vi "zlgcan_demo_I.vi"() -> ()   [LabVIEW 2013]
doc: "适用的设备：USBCAN-I、USBCAN-II、PCI9810、\nPCI9820、PCI5110、PCIe-9110I、PCI9820I、PCIE-9221、\nPCIe-9120I、PCI5121。"
uses:
  data_type/ZCAN_Transmit_Data.ctl
  data_type/ZCAN_InitCAN_setting_I.ctl
panel:
  in  "开启CAN":bool
  in  "I系列初始化参数":T1
  in  "stop":bool
  in  "?":T2(tab)
  in  "CAN 通道":u32(ring) items=["0", "1"]
  in  "CAN卡型号":u32(ring)=4 items=["PCI5121"=1, "PCI9810"=2, "USBCAN-I"=3, "USBCAN-II"=4, "PCI9820"=5, "PCI5110"=7, "CANET-UDP"=12, "PCI9840B"=14, "PCI9820I"=16, "CANET-TCP"=17, "PCIE9221"=24, "PCI-5010-U"=19, "PCI-5020-U"=22, "USBCAN_E_U"=20, "USBCAN_2E_U"=21, "USBCAN-4E-U"=31, "USBCAN-8E-U"=34, "PCIE-CANFD-400U"=40, "PCIE-CANFD-200U"=39, "PCIE-CANFD-100U"=38, "USBCANFD-200U"=41, "USBCANFD-100U"=42, "USBCANFD-MINI"=43, "PCIE-9120I"=27, "PCIE-9110I"=28, "PCIE-9140I"=29, "CANDTU-MINI"=33, "CANDTU-200 XX"=32]
  in  "索引":u32(ring) items=["0", "1", "2", "3", "4", "5", "6", "7", "8"]
  in  "波特率":u32(ring)=500000 items=["1Mbps"=1000000, "800kbps"=800000, "500kbps"=500000, "250kbps"=250000, "125kbps"=125000, "100kbps"=100000, "50kbps"=50000]
  in  "自定义波特率？":bool
  in  "自定义波特率字符输入":string
  in  "屏蔽码":u32=4294967295 format="%x"
  in  "工作模式":u8(ring) items=["正常", "只听"]
  in  "滤波模式":u8(ring) items=["双滤波", "单滤波"]
  in  "验收码":u32
  out "设备句柄":u32
  out "通道句柄":u32
  out "error out":errorcluster caption="状态"
  in  "帧类型":u32(ring) items=["标准帧", "扩展帧"]
  in  "发送方式":u32(ring) items=["正常发送", "单次发送", "自发自收", "单次自发自收"]
  in  "帧格式":u32(ring) items=["数据帧", "远程帧"]
  out "数据长度":u8=8 max=8
  in  "ID":u32=18 format="0x%08x"
  in  "协议":u32(ring) items=["CAN"]
  in  "数据输入":string="11 22 33 44 55 66 77 88"
  in  "发送":bool
  in  "CAN数据帧数组":T3(array[cluster])
  out "CAN报文显示":string[][](table)
  in  "ZCAN_Transmit_Data":T4
  out "已接收帧数":u32
  # "适用的设备：USBCAN-I、USBCAN-II、PCI9810、\nPCI9820、PCI5110、PCIe-9110I、PCI9820I、PCIE-9221、\nPCIe-9120I、PCI5121。"
  # "停止程序前，\n请先关闭CAN卡"
  # "1. 调试运行DEMO前，将bin文件夹下面的kerneldlls文件夹先拷贝至LabView安装目录，\n如 D:\\Program Files (x86)\\National Instruments\\LabVIEW 2018。"
  # "2. 确保电脑有VC++ 2005/2008/2010/2013运行库（对应32，64位），可到微软官网下载。"
  # "3，如果打开设备失败，可能原因：\n（1）没有进行第二步操作；\n（2）已经打开过一次，没有正常关闭的情况下，继续点击“打开设备”，是无法打开的。\n     需要USB重新拔插，LABVIEW重启（全部关闭），然后再“打开设备”。\n (3) 项目路径不能有中文繁体。"
  # "（默认可以不设置）"
  # "使用ZCANPro软件波特率计算工具计算"
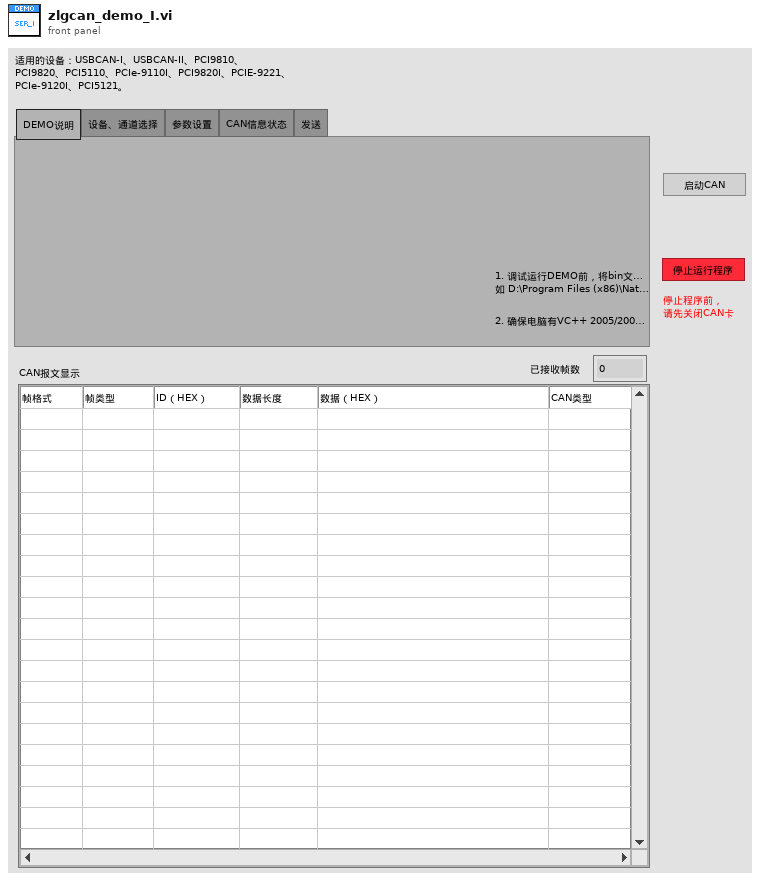
[diagram p1: front panel]
types:
  T1 = typedef "ZCAN_InitCAN_setting_I.ctl" = cluster{"baudrate":u32, "baud_rate_custom？":bool, "RateCustom":string, "filter":u8, "acc_code":u32, "acc_mask":u32, "mode":u8}
  T2 = enum32{"DEMO说明", "设备、通道选择", "参数设置", "CAN信息状态", "发送"}
  T3 = cluster{u32, u8, u8, u8, u8, cluster{"[0]":u8, "[1]":u8, "[2]":u8, "[3]":u8, "[4]":u8, "[5]":u8, "[6]":u8, "[7]":u8}, u64}[]
  T4 = typedef "ZCAN_Transmit_Data.ctl" = cluster{"帧类型":u32, "帧格式":u32, "ID":u32, "数据长度":u8, "DATA":cluster{"CAN数据[0]":u8, "CAN数据[1]":u8, "CAN数据[2]":u8, "CAN数据[3]":u8, "CAN数据[4]":u8, "CAN数据[5]":u8, "CAN数据[6]":u8, "CAN数据[7]":u8}, "发送方式":u32}
  T5 = cluster{"[0]":u32, "[1]":u32, "[2]":u32, "[3]":u32, "[4]":u32, "[5]":u32, "[6]":u32, "[7]":u32}
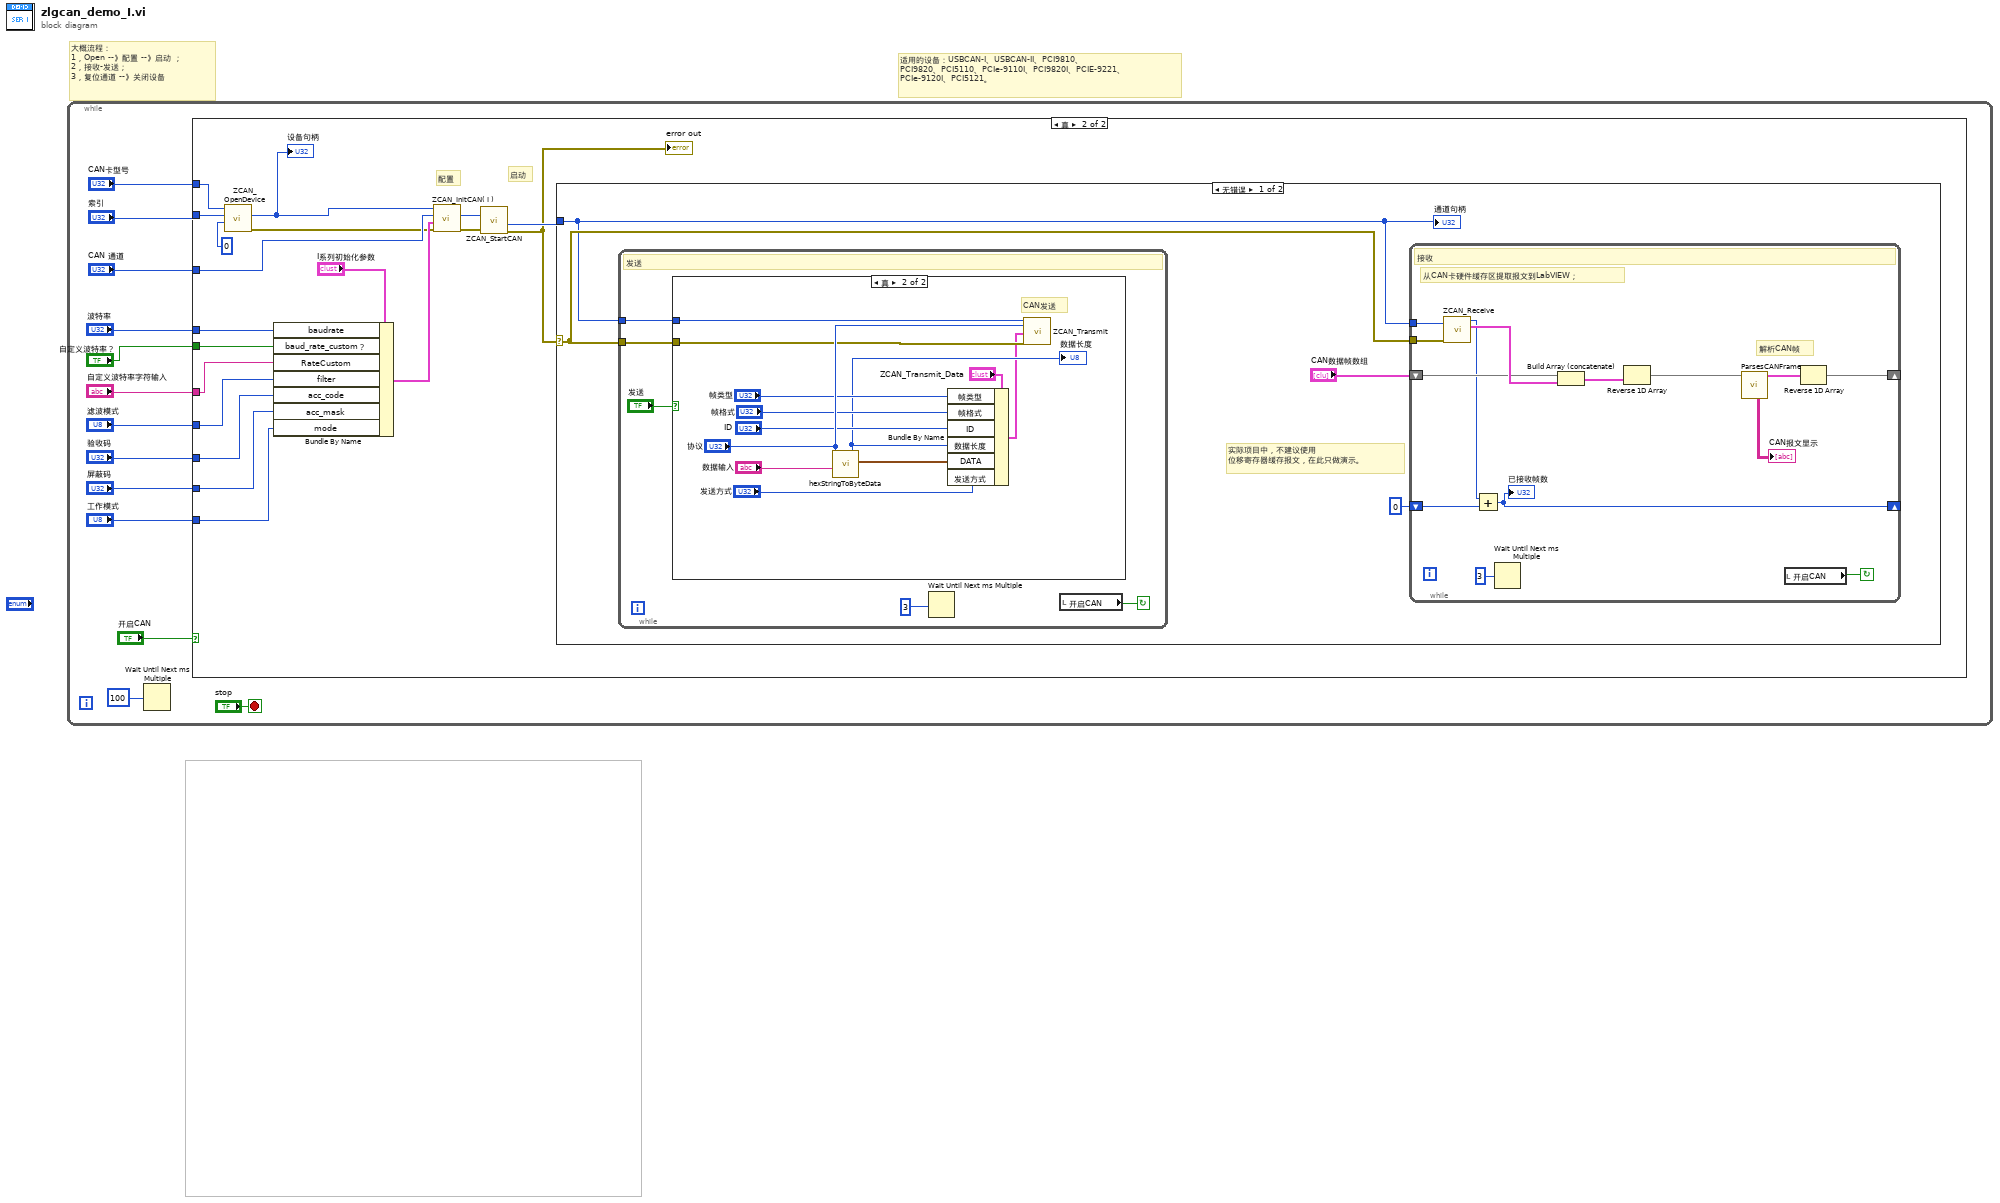
[diagram p0: block diagram]
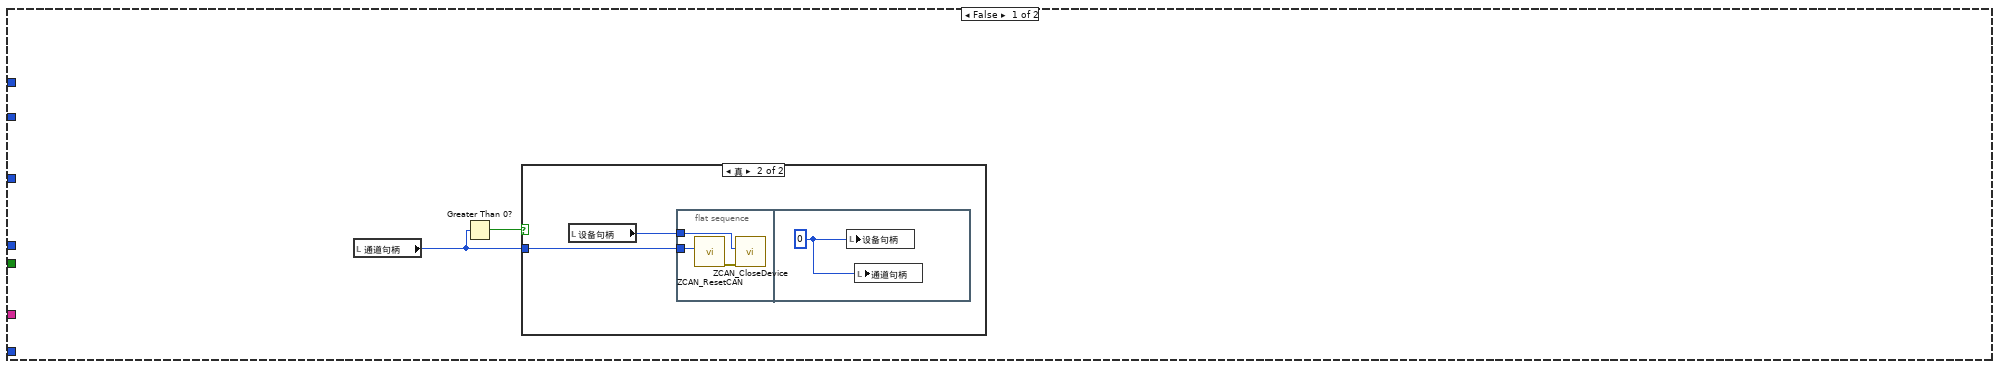
[diagram p2: hidden frame]
diagram:
  # "适用的设备：USBCAN-I、USBCAN-II、PCI9810、\nPCI9820、PCI5110、PCIe-9110I、PCI9820I、PCIE-9221、\nPCIe-9120I、PCI5121。"
  # "大概流程：\n1，Open --》配置 --》启动 ；\n2，接收-发送；\n3，复位通道 --》关闭设备"
  n1 = while {
    stop <- "stop" stop-if-true
    n2 = Wait Until Next ms Multiple(millisecond multiple=u32 100) -> ()  [unwired: 1 out]
    n3 = case shown="真" "开启CAN" {
      tunnel: "CAN 通道" -> [_ w32]
      tunnel: "CAN卡型号" -> [_ w38]
      tunnel: "索引" -> [_ w39]
      tunnel: "波特率" -> [_ w30]
      tunnel: "自定义波特率？" -> [_ w29]
      tunnel: "自定义波特率字符输入" -> [_ w28]
      tunnel: "滤波模式" -> [_ w27]
      tunnel: "验收码" -> [_ w26]
      tunnel: "屏蔽码" -> [_ w25]
      tunnel: "工作模式" -> [_ w24]
      frame False {
        # "关闭CAN卡"
        n4 = local read "通道句柄"() -> (w14:u32)
        n5 = Greater Than 0?(x=w14) -> (x > 0?=w15:bool)
        n6 = case shown="真" w15 {
          tunnel: w14 -> [_ w17]
          frame False {
          }
          frame True {
            n7 = local read "设备句柄"() -> (w16:u32)
            n8 = flat-sequence {
              tunnel: w17 -> [w19]
              tunnel: w16 -> [w18]
              frame #0 {
                n9 = call "ZCAN_ResetCAN.vi"("can_handle"=w19) -> ("error out"=w20:errorcluster)  [unwired: 9 in, 1 out]
                n10 = call "ZCAN_CloseDevice.vi"("error in (no error)"=w20, "device_handle"=w18) -> ()  [unwired: 8 in, 2 out]
              }
              frame #1 {
                w21 = u32 0 ("can_index_handle(out)")
                n11 = local write "设备句柄"(w21) -> ()
                n12 = local write "通道句柄"(w21) -> ()
              }
            }
          }
        }
      }
      frame True {
        # "启动"
        # "配置"
        n13 = call "ZCAN_OpenDevice.vi"("reserved"=0, "device_index"=w39, "device_type"=w38) -> ("error out"=w22:errorcluster, "DEVICE_HANDLE"=w23:u32)  [unwired: 7 in]
        "设备句柄" <- w23
        n14 = Bundle By Name(cluster="I系列初始化参数", "baudrate"=w30, "baud_rate_custom？"=w29, "RateCustom"=w28, "filter"=w27, "acc_code"=w26, "acc_mask"=w25, "mode"=w24) -> (w34:T1)
        n15 = call "ZCAN_InitCAN( I ).vi"("error in (no error)"=w22, "I系列初始化参数"=w34, "can_index"=w32, "device_hande"=w23) -> ("error out"=w33:errorcluster, "can_index_handle"=w31:u32)  [unwired: 2 in]
        n16 = call "ZCAN_StartCAN.vi"("error in (no error)"=w33, "can_index_handle"=w31) -> ("error out"=w36:errorcluster, "can_index_handle(out)"=w37:u32)  [unwired: 7 in, 1 out]
        "error out" <- w36
        n17 = case shown="无错误" w36 {
          selector: w36 -> [w43 _]
          tunnel: w37 -> [w42 _]
          frame No Error {
            # "实际项目中，不建议使用\n位移寄存器缓存报文，在此只做演示。"
            n18 = while {
              tunnel: w42 -> [w61]
              tunnel: w43 -> [w59]
              stop <- w60 continue-if-true
              # "发送"
              n19 = case shown="真" "发送" {
                tunnel: w61 -> [_ w68]
                tunnel: w59 -> [_ w69]
                frame False {
                }
                frame True {
                  # "CAN发送"
                  n20 = call "hexStringToByteData.vi"("数据输入"="数据输入", "协议"="协议") -> ("CAN_data"=w65:T5, "字节数"=w70:i32)  [unwired: 7 in, 1 out]
                  "数据长度" <- w70
                  n21 = Bundle By Name(cluster="ZCAN_Transmit_Data", "帧类型"="帧类型", "帧格式"="帧格式", "ID"="ID", "数据长度"=w70, "DATA"=w65, "发送方式"="发送方式") -> (w64:T4)
                  n22 = call "ZCAN_Transmit.vi"("can_index_handle"=w68, "协议"="协议", "ZCAN_Transmit_Data"=w64, "error in (no error)"=w69) -> ()  [unwired: 15 in, 1 out]
                }
              }
              n23 = Wait Until Next ms Multiple(millisecond multiple=u32 3) -> ()  [unwired: 1 out]
              n24 = local read "开启CAN"() -> (w60:bool)
            }
            n25 = while {
              tunnel: w43 -> [w56]
              tunnel: w42 -> [w55]
              shift-right: [w57] -> _
              shift-left: 0 -> [w46]
              shift-right: [w49] -> _
              shift-left: "CAN数据帧数组" -> [w52]
              stop <- w54 continue-if-true
              # "从CAN卡硬件缓存区提取报文到LabVIEW；"
              # "解析CAN帧"
              # "接收"
              n26 = call "ZCAN_Receive.vi"("error in (no error)"=w56, "can_handle"=w55) -> ("CAN数据帧数组"=w53:T3, "Receive_Num"=w47:u32)  [unwired: 2 in, 2 out]
              n27 = Add(x=w47, y=w46) -> (x+y=w57:u32)
              "已接收帧数" <- w57
              n28 = Wait Until Next ms Multiple(millisecond multiple=u32 3) -> ()  [unwired: 1 out]
              n29 = Build Array (concatenate)(w52, w53) -> (w51:T3)
              n30 = Reverse 1D Array(array=w51) -> (reversed array=w48:T3)
              n31 = call "ParsesCANFrame.vi"("CAN数据帧数组"=w48) -> ("CAN数据帧数组(out)"=w50:T3, "CAN报文显示"=→"CAN报文显示":string[][])  [unwired: 9 in]
              n32 = local read "开启CAN"() -> (w54:bool)
              n33 = Reverse 1D Array(array=w50) -> (reversed array=w49:T3)
            }
            "通道句柄" <- w42
          }
          frame Error {
          }
        }
      }
    }
  }
